vi "mysql读取.vi"() -> ()   [LabVIEW 2020]
uses:
  <vilib>/addons/database/Connection.llb/DB Tools Open Connec (Path).vi
  <vilib>/addons/database/Connection.llb/Conn Execute.vi
  <vilib>/addons/database/Recordset.llb/Rec Fetch Recordset Data (R).vi
  <vilib>/addons/database/Recordset.llb/Rec Destroy - Connection.vi
  <vilib>/addons/database/_DB Variant To Data/Database Variant To Data.xnode
  <vilib>/addons/database/NI_Database_API.lvlib
panel:
  out "元素":variant
  out "email值":string
  out "转化为字符串":string
  out "error out":errorcluster
  in  "connection information":path
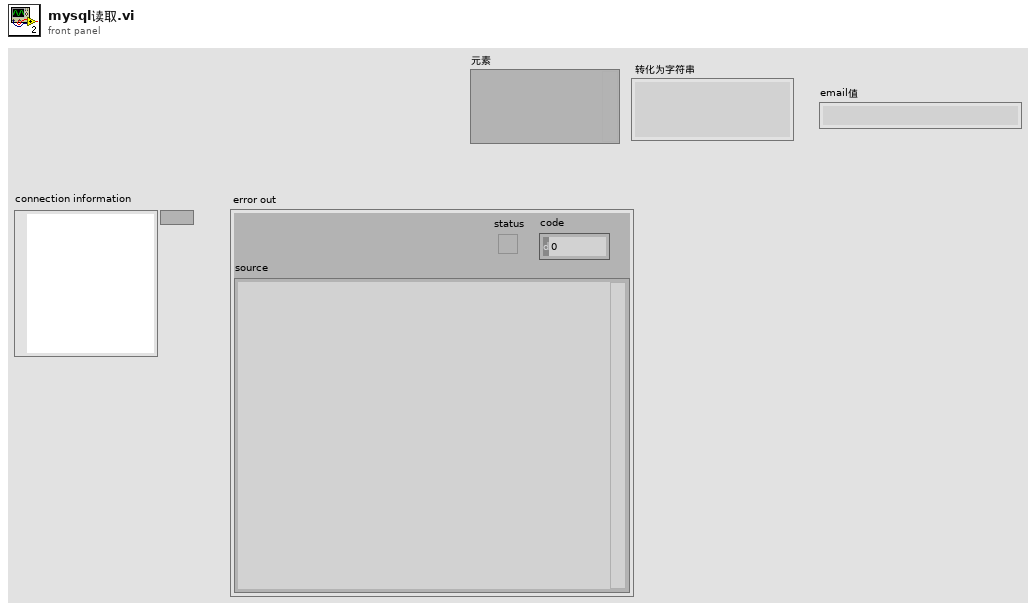
[diagram p1: front panel]
types:
  T1 = typedef "NI_Database_API.lvlib/Conn ObjectReference.ctl" = refnum<k1>
  T2 = typedef "NI_Database_API.lvlib/Rec ObjectReference.ctl" = refnum<k1>
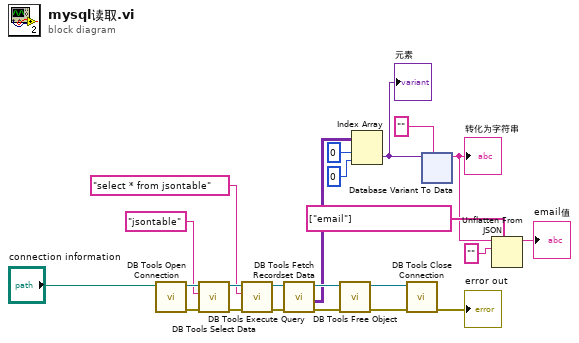
[diagram p0: block diagram]
diagram:
  n1 = call-poly <vilib>:"DB Tools Open Connection.vi"("connection information"="connection information") -> ("error out"=w22:errorcluster, "connection reference"=w21:T1)  [unwired: 7 in]
  n2 = call <vilib>:"DB Tools Select Data.vi"("error in (no error)"=w22, "table"="jsontable", "connection reference"=w21) -> ("error out"=w2:errorcluster, "connection reference out"=w19:T1)  [unwired: 3 in, 1 out]
  n3 = call-poly <vilib>:"DB Tools Execute Query.vi"("error in (no error)"=w2, "SQL query"="select * from jsontable", "connection reference"=w19) -> ("error out"=w11:errorcluster, "recordset reference"=w1:T2)  [unwired: 5 in]
  n4 = call-poly <vilib>:"DB Tools Fetch Recordset Data.vi"("error in (no error)"=w11, "recordset reference"=w1) -> ("error out"=w10:errorcluster, "recordset data"=w4:variant[][], "recordset reference out"=w13:T2)  [unwired: 3 in]
  n5 = call-poly <vilib>:"DB Tools Free Object.vi"("error in (no error)"=w10, "recordset reference"=w13) -> ("error out"=w9:errorcluster, "connection reference"=w12:T1)  [unwired: 8 in]
  n6 = Index Array(array=w4, index (row)=0 ("索引 (行)"), index (col)=0 ("禁用的索引 (列)")) -> (element=w15:variant)
  "元素" <- w15
  n7 = call <vilib>:"DB Tools Close Connection.vi"("error in (no error)"=w9, "connection reference"=w12) -> ("error out"=→"error out":errorcluster)  [unwired: 5 in]
  n8 = xnode "Database Variant To Data"("database variant"=w15, "type"="") -> ("data"=w3:string)  [unwired: 1 in, 1 out]
  "转化为字符串" <- w3
  n9 = Unflatten From JSON(path=string[] ["email"] ("路径"), JSON string=w3, type and defaults="") -> (value=→"email值":string)  [unwired: 4 in, 1 out]
